vi "Upgrade Firmware.vi"   [LabVIEW 2014, in "nisyscfg.lvlib"]
doc: "Updates the firmware on the target. You can specify to update a file or the version."
uses:
  nisyscfg.lvlib
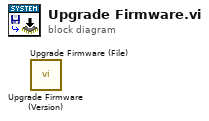
[diagram p0: block diagram]
diagram:
  n1 = call "Upgrade Firmware (Version).vi"() -> ()  [unwired: 8 in, 4 out]
  n2 = call "Upgrade Firmware (File).vi"() -> ()  [unwired: 8 in, 4 out]
